vi "Check Clicked Item.vi"(7 "error in (no error)":errorcluster, 10 "Affected Items":T2) -> (0 "error out":errorcluster, 2 "Type":T1, 3 "Type Definition/Class Path":string, 4 "Typedef/Class Data?":bool)   [LabVIEW 2020]
uses:
  7ec5ad4a-e670-451f-9999-370eac425bf5.vi
  95405c5a-1f30-4ca8-8e6e-823794fec552.vi
  003fbabe-b691-4ee5-81d2-41f7bedf5711.vi
  OpenTypeDef-RunTime.ctl
  <vilib>/Utility/Data Type/Type Definitions/Data Type.ctl
  <vilib>/Utility/Data Type/NI_Data Type.lvlib
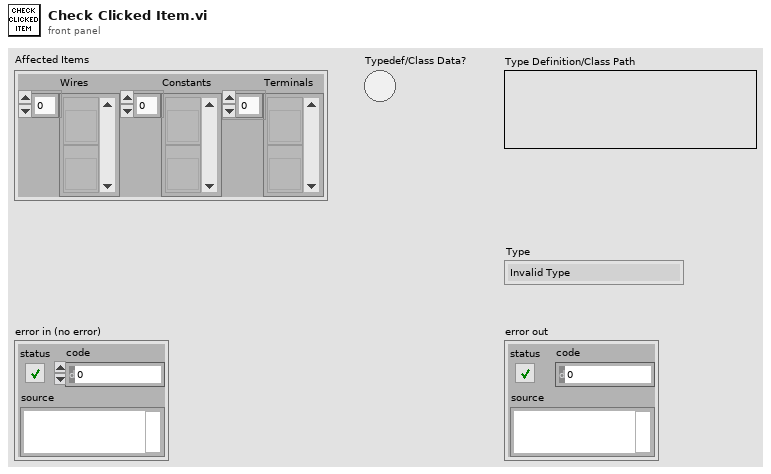
[diagram p1: front panel]
types:
  T1 = typedef "NI_Data Type.lvlib/Data Type.ctl" = enum8{"Invalid Type", "Void", "I8", "I16", "I32", "I64", "U8", "U16", "U32", "U64", "Single Float", "Double Float", "Extended Float", "Single Complex", "Double Complex", "Extended Complex", "Enum U8", "Enum U16", "Enum U32", "Enum U64", "Single Float With Unit", "Double Float With Unit", "Extended Float With Unit", "Single Complex with Unit", "Double Complex with Unit", "Extended Complex with Unit", "Boolean", "String", "Path", "Picture", "Tag", "Array", "Cluster", "Variant", "LV Variant", "Waveform", "Timestamp", "Digital Waveform", "Digital Data", "ExpressData", "Refnum", "External Data", "VI", "Poly VI", "LabVIEW Class Instance", "Fixed Point", "Set Collection", "Map Collection"}
  T2 = typedef "OpenTypeDef-RunTime.ctl" = cluster{"Wires":refnum<vi>[], "Constants":refnum<vi>[], "Terminals":refnum<vi>[]}
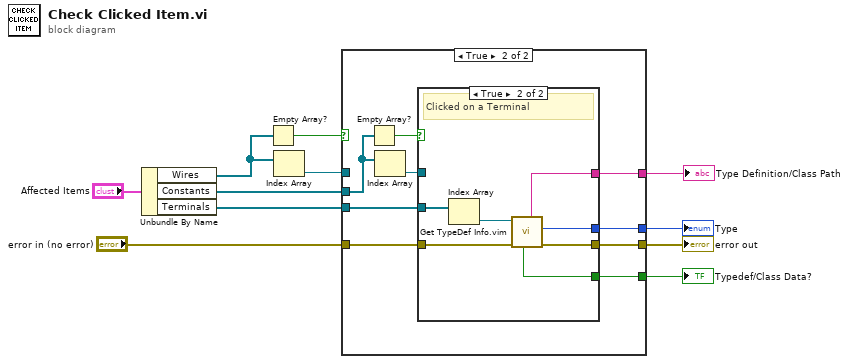
[diagram p0: block diagram]
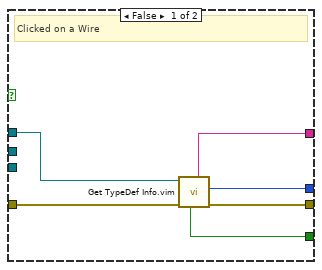
[diagram p2: hidden frame]
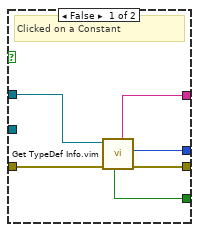
[diagram p3: hidden frame]
diagram:
  n1 = Unbundle By Name("Affected Items") -> ("Wires"=w7:refnum<vi>[], "Constants"=w10:refnum<vi>[], "Terminals"=w9:refnum<vi>[])
  n2 = Empty Array?(array=w7) -> (empty?=w8:bool)
  n3 = Index Array(array=w7) -> (element=w6:refnum<vi>)  [unwired: 1 in]
  n4 = case shown="True" w8 {
    tunnel: w10 -> [_ w26]
    tunnel: w9 -> [_ w25]
    tunnel: w6 -> [w12 _]
    tunnel: "error in (no error)" -> [w17 w22]
    tunnel: [w16 w21] -> w4
    tunnel: [w15 w18] -> w3
    tunnel: [w14 w19] -> w2
    tunnel: [w13 w20] -> w1
    frame False {
      # "Clicked on a Wire"
      n5 = call "Get TypeDef Info.vim"("error in (no error)"=w17, "Ref in"=w12) -> ("error out"=w16:errorcluster, "Type"=w15:T1, "Type Definition/Class Path"=w14:string, "Typedef/Class Data?"=w13:bool)  [unwired: 3 in, 1 out]
    }
    frame True {
      n6 = Empty Array?(array=w26) -> (empty?=w24:bool)
      n7 = Index Array(array=w26) -> (element=w23:refnum<vi>)  [unwired: 1 in]
      n8 = case shown="True" w24 {
        tunnel: w25 -> [_ w39]
        tunnel: w23 -> [w30 _]
        tunnel: w22 -> [w32 w34]
        tunnel: [w31 w38] -> w21
        tunnel: [w29 w35] -> w20
        tunnel: [w28 w36] -> w19
        tunnel: [w27 w37] -> w18
        frame False {
          # "Clicked on a Constant"
          n9 = call "Get TypeDef Info.vim"("error in (no error)"=w32, "Ref in"=w30) -> ("error out"=w31:errorcluster, "Type"=w27:T1, "Type Definition/Class Path"=w28:string, "Typedef/Class Data?"=w29:bool)  [unwired: 3 in, 1 out]
        }
        frame True {
          # "Clicked on a Terminal"
          n10 = Index Array(array=w39) -> (element=w33:refnum<vi>)  [unwired: 1 in]
          n11 = call "Get TypeDef Info.vim"("error in (no error)"=w34, "Ref in"=w33) -> ("error out"=w38:errorcluster, "Type"=w37:T1, "Type Definition/Class Path"=w36:string, "Typedef/Class Data?"=w35:bool)  [unwired: 3 in, 1 out]
        }
      }
    }
  }
  "error out" <- w4
  "Typedef/Class Data?" <- w1
  "Type Definition/Class Path" <- w2
  "Type" <- w3
